vi "Copy .LLB to NI VeriStand dir.vi"(5 "Files Generated by Build":path[](array[path]), 6 "Top Level/Always Included VIs":path[](array[path]), 7 "Destination Path":path, 8 "error in (no error)":errorcluster, 9 "Target Name":string, 10 "Build Specification Name":string, 11 "Project Path":path) -> (0 "error out":errorcluster)   [LabVIEW 2027]
doc: "This VI is called after each run of a build specification. The VI will copy the generated LLB (Engine or System Explorer) into the VeriStand Custom Device folder (...\\Documents\\National Instruments\\NI VeriStand 2013...)."
uses:
  <vilib>/Utility/sysdir.llb/System Directory Type.ctl
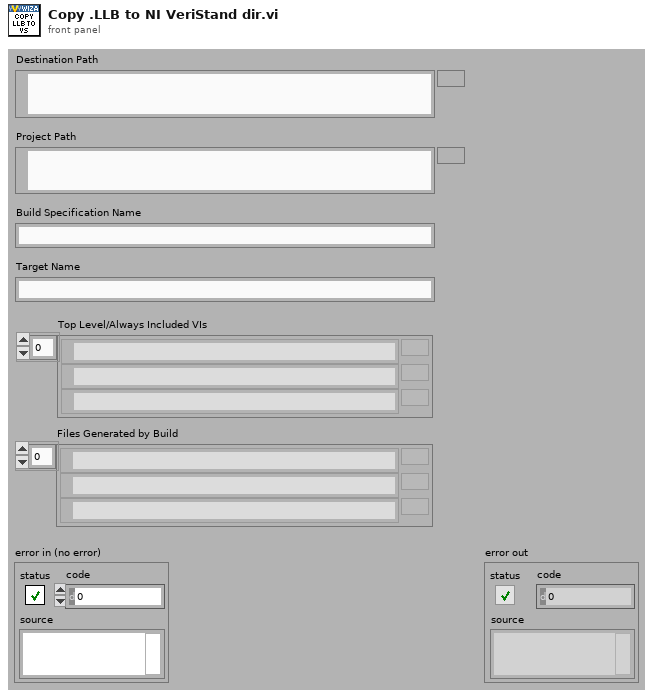
[diagram p1: front panel]
types:
  T1 = typedef "System Directory Type.ctl" = i32
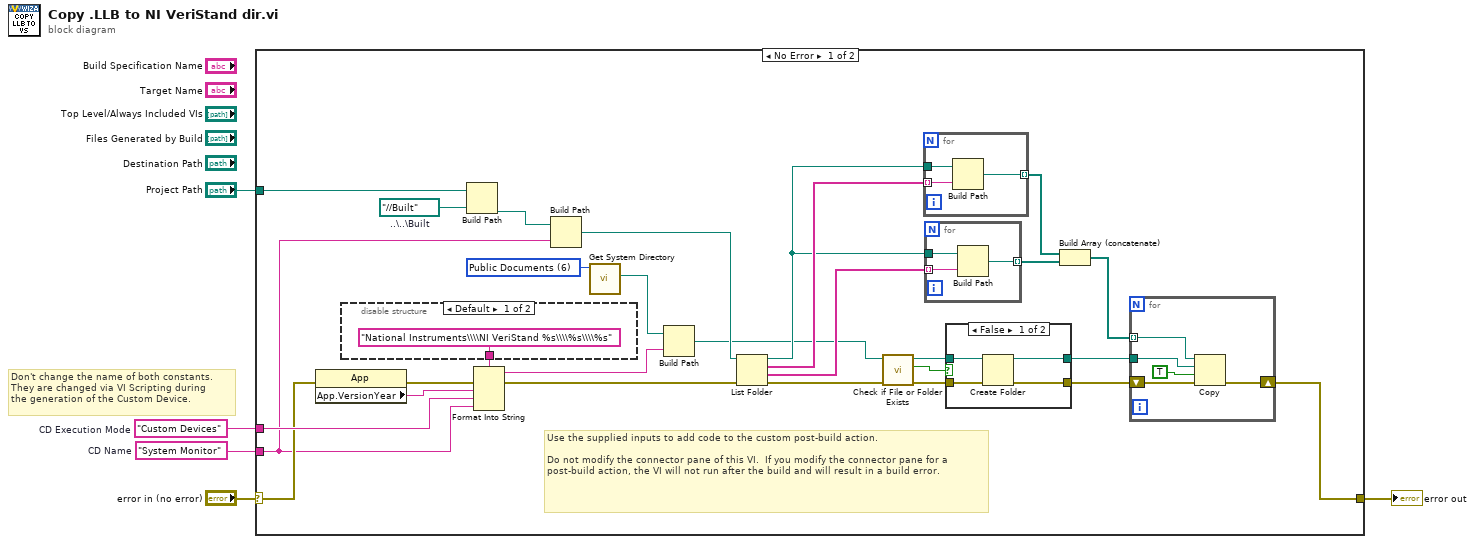
[diagram p0: block diagram]
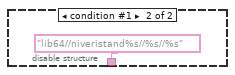
[diagram p2: hidden frame]
diagram:
  w2 = "System Monitor"  # CD Name
  w3 = "Custom Devices"  # CD Execution Mode
  # "Don't change the name of both constants.\nThey are changed via VI Scripting during\nthe generation of the Custom Device."
  n1 = case shown="No Error" "error in (no error)" {
    selector: "error in (no error)" -> [w12 w53]
    tunnel: [w15 w53] -> w1
    tunnel: "Project Path" -> [w9 _]
    tunnel: w3 -> [w13 _]
    tunnel: w2 -> [w10 _]
    frame No Error {
      w6 = path "../../Built"  # ..\..\Built
      w19 = T1 6 items=["User Home"=0, "User Desktop"=1, "User Documents"=2, "User Application Data"=3, "User Preferences"=4, "User Temporary"=5, "Public Documents"=6, "Public Application Data"=7, "Public Preferences"=8, "Public Cache"=13, "System Core Libraries"=9, "System Installed Libraries"=10, "Application Files"=11, "Boot Volume Root"=12] ("system directory type")
      # "Use the supplied inputs to add code to the custom post-build action.\n\nDo not modify the connector pane of this VI.  If you modify the connector pane for a post-build action, the VI will not run after the build and will result in a build error."
      n2 = property class="App"(error in=w12) -> (error out=w18:errorcluster, "App.VersionYear"=w17:string)  [unwired: 1 in, 1 out]
      n3 = disable-structure shown="Default" {
        disable-tunnel: ["National Instruments\\\\NI VeriStand %s\\\\%s\\\\%s" ("name or relative path") "lib64//niveristand%s//%s//%s" ("name or relative path")] -> w16
        frame condition #0 (active) {
        }
        frame condition #1 {
        }
      }
      n4 = Build Path(base path=w9, name or relative path=w6) -> (appended path=w22:path)
      n5 = Format Into String(format string=w16, error in=w18, w17, w13, w10) -> (resulting string=w21:string, error out=w11:errorcluster)  [unwired: 1 in]
      n6 = Build Path(base path=w22, name or relative path=w10) -> (appended path=w24:path)
      n7 = call <vilib>:"Get System Directory.vi"("system directory type"=w19) -> ("system directory"=w20:path)  [unwired: 10 in]
      n8 = Build Path(base path=w20, name or relative path=w21) -> (appended path=w14:path)
      n9 = List Folder(path=w24, error in=w11) -> (path out=w26:path, filenames=w33:string[], folder names=w27:string[], error out=w23:errorcluster)  [unwired: 2 in]
      n10 = call <vilib>:"Check if File or Folder Exists.vi"("error in (no error)"=w23, "path"=w14) -> ("error out"=w28:errorcluster, "file or folder exists?"=w30:bool, "dup path"=w29:path)  [unwired: 7 in]
      n11 = for {
        tunnel: w33 -> [w51] mode=indexing
        tunnel: w26 -> [w52]
        tunnel: [w50] -> w32 mode=indexing
        n12 = Build Path(base path=w52, name or relative path=w51) -> (appended path=w50:path)
      }
      n13 = for {
        tunnel: w27 -> [w48] mode=indexing
        tunnel: w26 -> [w49]
        tunnel: [w47] -> w25 mode=indexing
        n14 = Build Path(base path=w49, name or relative path=w48) -> (appended path=w47:path)
      }
      n15 = case shown="False" w30 {
        tunnel: w29 -> [w39 w41]
        tunnel: w28 -> [w38 w40]
        tunnel: [w37 w41] -> w8
        tunnel: [w36 w40] -> w7
        frame False {
          n16 = Create Folder(path (use dialog)=w39, error in=w38) -> (created path=w37:path, error out=w36:errorcluster)  [unwired: 1 in, 1 out]
        }
        frame True {
        }
      }
      n17 = Build Array (concatenate)(w32, w25) -> (w31:path[])
      n18 = for {
        tunnel: w31 -> [w43] mode=indexing
        shift-right: [w44] -> w15
        shift-left: w7 -> [w45]
        tunnel: w8 -> [w42]
        n19 = Copy(8:w45, 9:TRUE ("overwrite (F)"), 10:w42, 11:w43) -> (0:w44:errorcluster)  [unwired: 1 in, 2 out]
      }
    }
    frame Error {
    }
  }
  "error out" <- w1
